vi "VersionDialog(CSM).vi"(7 "Name (\"\" to Use UUID)":string="Event CSM Tiny") -> ()   [LabVIEW 2020, in "CSMStand(Lite).lvlib"]
doc: "------------- lvcsm -------------\n[CSMStates]\nItem 0 = \"Event Structure\"\nItem 1 = \"Idle\"\nItem 2 = \"CSM Documentation\"\nItem 3 = \"VI Reference\"\nItem 4 = \"Error Handler\"\nItem 5 = \"Critical Error\"\nItem 6 = \"Target Error\"\nItem 7 = \"Target Timeout Error\"\nItem 8 = \"Async Response\"\nItem 9 = \"Response\"\nItem 10 = \"Async Message Posted\"\nItem 11 = \"Initialize Core Data\"\nItem 12 = \"Exit\"\nItem 13 = \"Data: Initialize\"\nItem 14 = \"Data: Cleanup\"\nItem 15 = \"Events: Register\"\nItem 16 = \"Events: Unregister\"\nItem 17 = \"UI: Initialize\"\nItem 18 = \"UI: Cursor Set\"\nItem 19 = \"UI: Front Panel State\"\nItem 20 = \"Macro: Initialize\"\nItem 21 = \"Macro: Exit\"\nItem 22 = \"API: API1\"\nItem 23 = \"API: API2\"\nItem 24 = \"Action: action1\"\nItem 25 = \"Action: action2\"\n\n[CSMStatus]\nItem 0 = \"Error Occurred@Error Handler\""
uses:
  CSMStand(Lite).lvlib
  <userlib>/_NEVSTOP/Communicable State Machine(CSM)/AdvanceAPI/CSM - Revert Arguments-Safe String.vi
  <userlib>/_NEVSTOP/Communicable State Machine(CSM)/AdvanceAPI/CSM - Make String Arguments Safe.vi
  <userlib>/_NEVSTOP/Communicable State Machine(CSM)/AdvanceAPI/CSM - Break Down Multiple States String.vi
  <userlib>/_NEVSTOP/Communicable State Machine(CSM)/AdvanceAPI/CSM - Compact Multiple States.vi
  <userlib>/_NEVSTOP/Communicable State Machine(CSM)/AdvanceAPI/CSM - Keywords.vi
  <userlib>/_NEVSTOP/Communicable State Machine(CSM)/_Shared/Trim Single-line Text.vi
  <userlib>/NEVSTOP-Programming-Palette/Dialog & Interface/Fit VI window to Visible Content_nevstop.vi
  <userlib>/_NEVSTOP/Communicable State Machine(CSM)/Communicable State Machine.lvlib
  <userlib>/_NEVSTOP/Communicable State Machine(CSM)/addons/API-String-Arugments-Support/API String Arguments Support.lvlib
panel:
  out "CSMVersion 2":string="Powered By CSM, Copyright ?2025 NEVSTOP-LAB"
  out "CSMStand(version) 2":string="CSMStand-Lite"
  out "CSMVersion":string
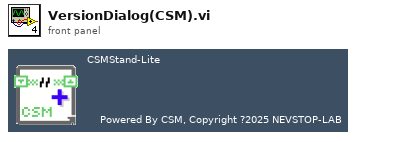
[diagram p1: front panel]
types:
  T1 = enum32{"Invalid", "Standard", "Closed", "Hidden", "Minimized", "Maximized"}
  T2 = enum32{"invalid app kind", "Development System", "Run Time System", "Student Edition", "Embedded LabVIEW", "Evaluation", "Custom"}
  T3 = typedef "Communicable State Machine.lvlib/_CSM_Response Source Message.ctl" = cluster{"‘State":string, "’Arguments":string, "’Error":errorcluster}
  T4 = cluster{"Current VI Reference":refnum<vi>, "Close Panel on Exit?":bool}
  T5 = cluster{"Core":cluster{"Current VI Reference":refnum<vi>, "Close Panel on Exit?":bool}, "Your Boolean data":bool, "Your string data":string}
  T6 = cluster{"Major":u16, "Minor":u16, "Fix":u16, "Build":u16}
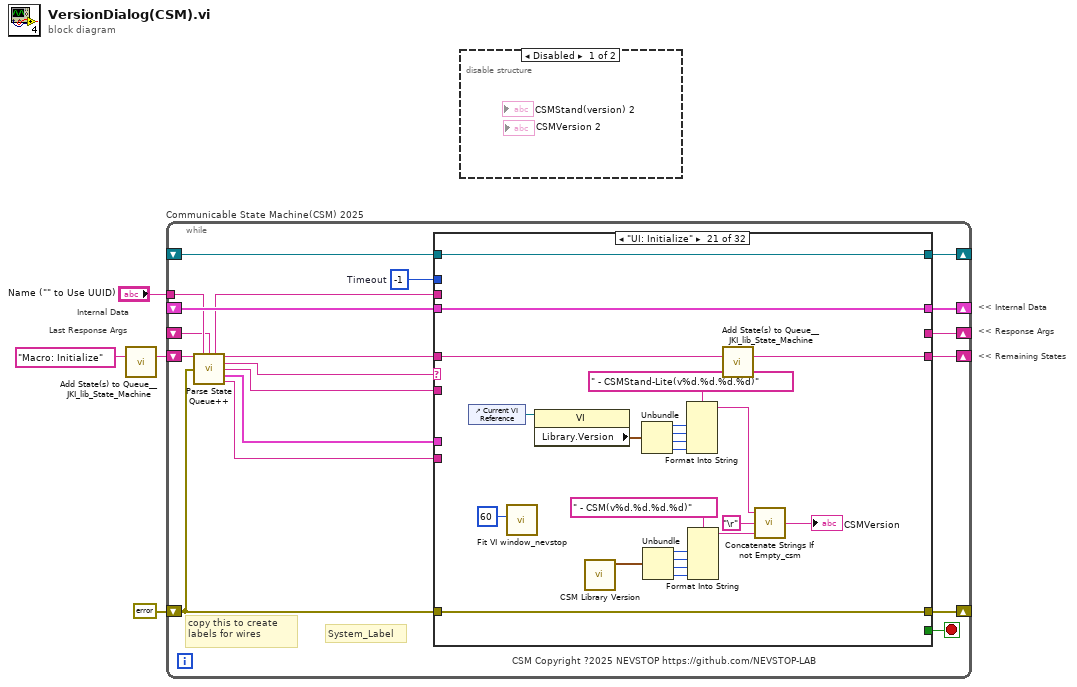
[diagram p0: block diagram]
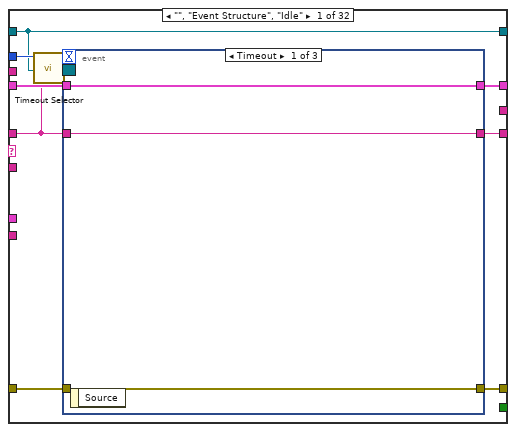
[diagram p3: hidden frame]
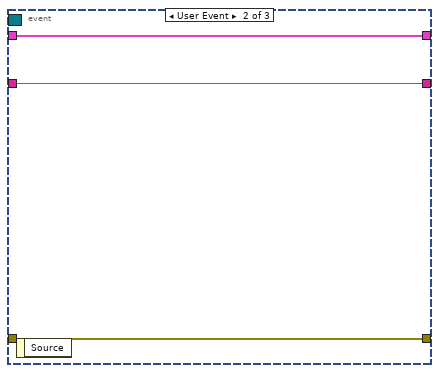
[diagram p4: hidden frame]
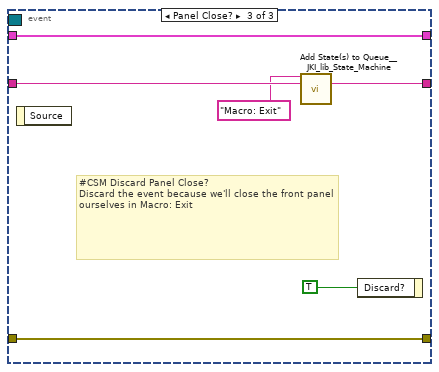
[diagram p5: hidden frame]
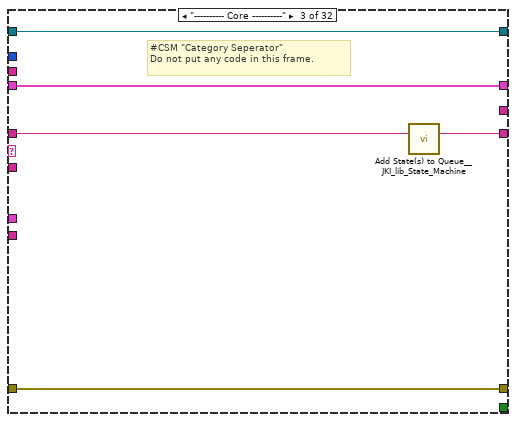
[diagram p7: hidden frame]
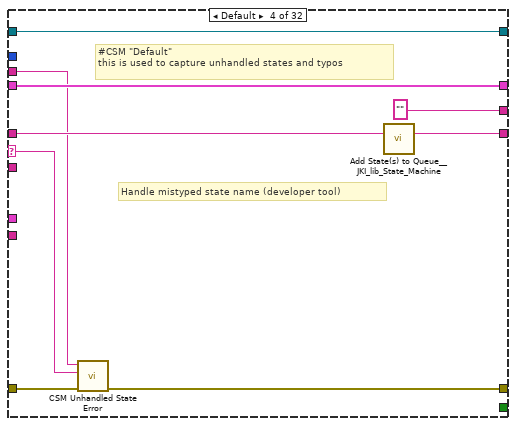
[diagram p8: hidden frame]
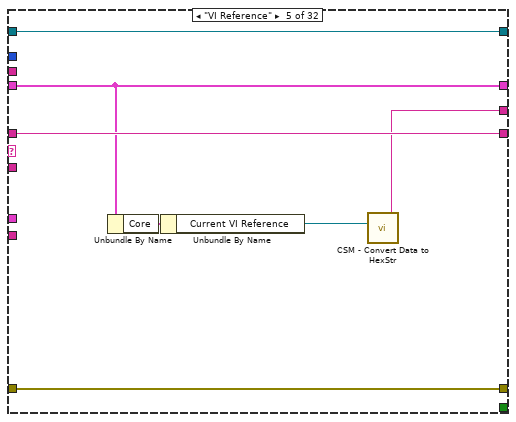
[diagram p9: hidden frame]
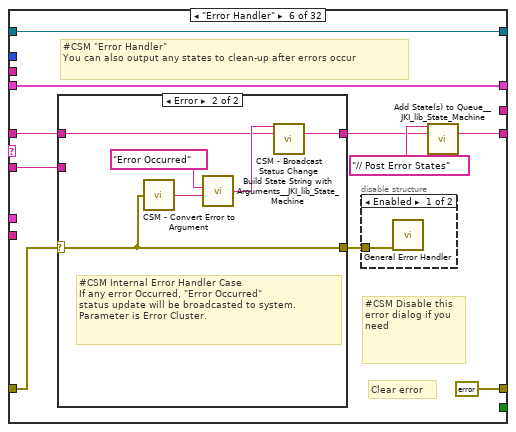
[diagram p10: hidden frame]
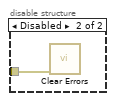
[diagram p11: hidden frame]
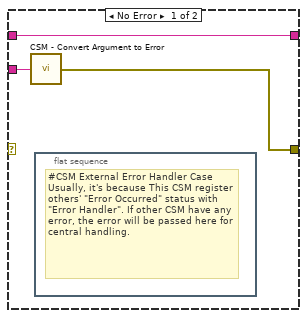
[diagram p12: hidden frame]
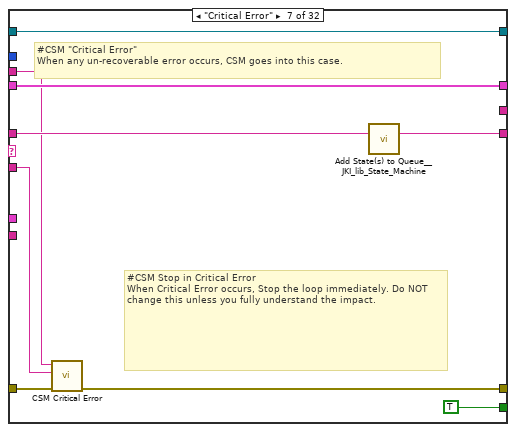
[diagram p13: hidden frame]
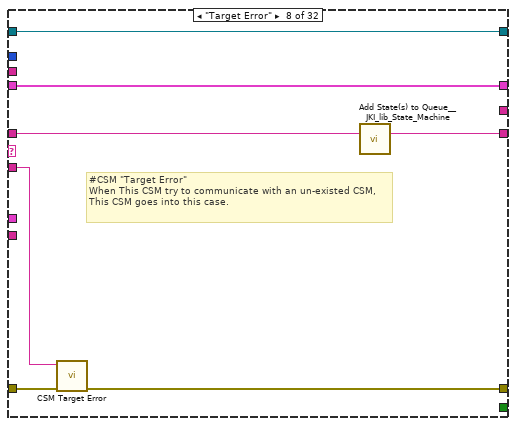
[diagram p14: hidden frame]
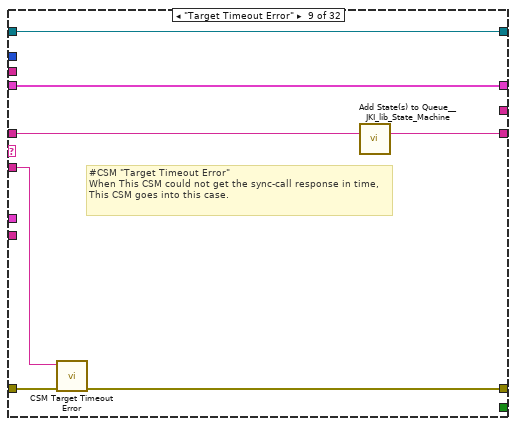
[diagram p15: hidden frame]
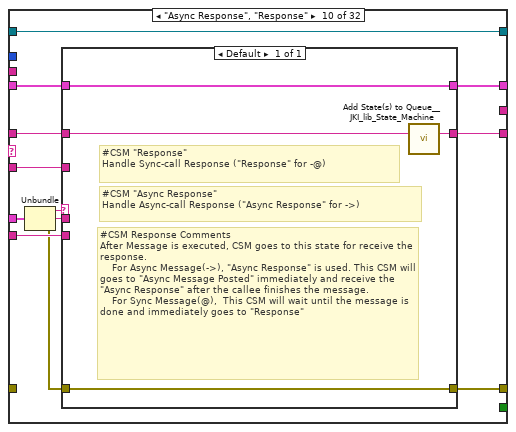
[diagram p16: hidden frame]
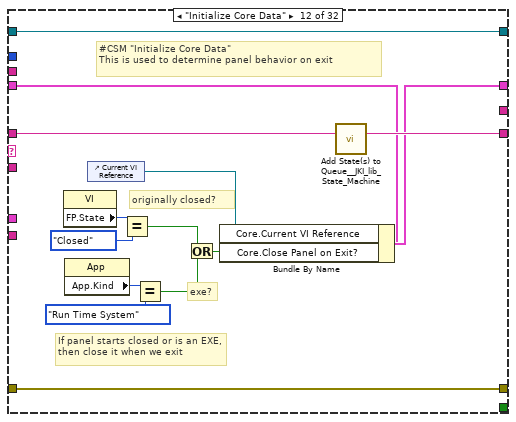
[diagram p18: hidden frame]
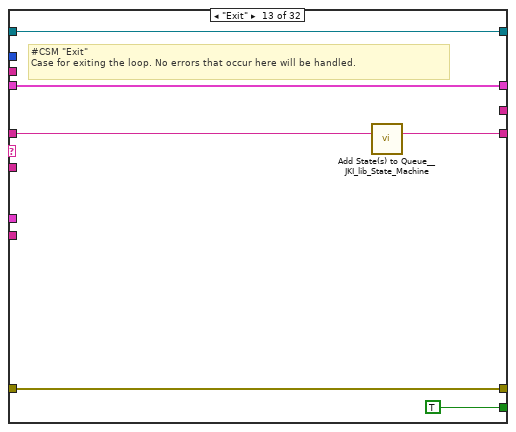
[diagram p19: hidden frame]
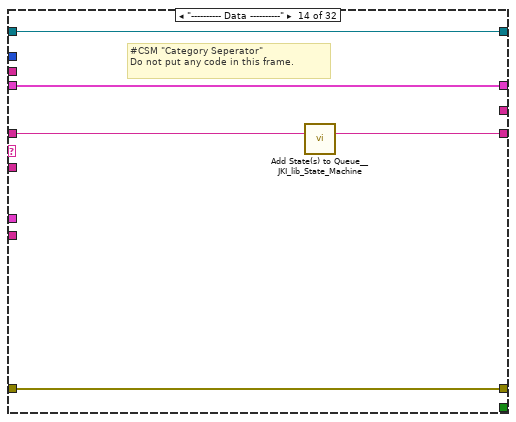
[diagram p20: hidden frame]
diagram:
  # "Last Response Args"
  # "Internal Data"
  # "<< Internal Data"
  # "<< Response Args"
  # "<< Remaining States"
  n1 = call <vilib>:"Add State(s) to Queue__JKI_lib_State_Machine.vi"("State(s) in (\"\")"="Macro: Initialize" ("Init State(\"Macro: Initialize\")")) -> ("States Out"=w1:string)  [unwired: 14 in]
  n2 = while "Communicable State Machine(CSM) 2025" {
    shift-right: [w18] -> _
    shift-left: _ -> [w17]
    shift-right: [w21] -> _
    shift-left: errorcluster {"status"=FALSE, "code"=0, "source"=""} ("error out") -> [w15]
    shift-right: [w20] -> _
    shift-left: w1 -> [w22]
    tunnel: "Name (\"\" to Use UUID)" -> [w11]
    shift-right: [w14] -> _
    shift-left: _ -> [w5]
    shift-right: [w13] -> _
    shift-left: _ -> [w12]
    stop <- w19 stop-if-true
    w16 = -1  # Timeout
    # "copy this to create labels for wires"
    # "System_Label"
    # "CSM Copyright ?2025 NEVSTOP https://github.com/NEVSTOP-LAB"
    n3 = call <userlib>:"Parse State Queue++.vi"("State Queue"=w22, "Name (\"\" to Use UUID)"=w11, "Response Arguments"=w5, "Previous Error"=w15) -> ("Name Used"=w6:string, "Remaining States"=w23:string, "Current State"=w10:string, "Arguments"=w9:string, "Additional Information"=w8:T3, "Source CSM"=w7:string)  [unwired: 6 in]
    n4 = case shown="\"UI: Initialize\"" w10 {
      selector: w10 -> [_ _ _ w56 _ _ _ _ _ _ _ _ _ _ _ _ _ _ _ _ _ _ _ _ _ _ _ _ _ _ _ _]
      tunnel: w23 -> [w24 w47 w53 w61 w68 w74 w97 w103 w110 w119 w132 w147 w153 w158 w166 w173 w178 w185 w189 w195 w218 w225 w241 w311 w317 w329 w332 w337 w343 w351 w356 w361]
      tunnel: w9 -> [_ _ _ _ _ w73 w92 w102 w109 w118 _ _ _ _ _ _ _ _ _ _ _ w220 w235 _ _ _ _ _ w340 _ _ _]
      tunnel: w17 -> [w31 w46 w50 w59 w67 w78 w98 w105 w112 w121 w131 w140 w151 w155 _ w168 w175 w184 w188 w192 w216 w223 w237 w308 w314 w326 w331 w336 w342 w348 w353 w358]
      tunnel: [w30 w48 w51 w54 w69 errorcluster {"status"=FALSE, "code"=0, "source"=""} ("error out") w93 w100 w107 w124 w133 w144 w150 w156 w163 w169 w176 w179 w187 w193 w215 w221 w238 w309 w315 w327 w333 w338 w344 w349 w354 w359] -> w21
      tunnel: w15 -> [w29 w48 w51 w62 w69 w75 w99 w101 w108 _ w133 w144 w150 w156 w163 w170 w176 _ w190 w193 w215 w222 w239 w309 w315 w327 w333 w338 w344 w349 w354 w359]
      tunnel: [w32 w47 w52 w60 w68 w70 w96 w106 w113 w120 w132 w146 w152 w157 w165 w172 w177 w185 w189 w194 w217 w224 w240 w310 w316 w328 w332 w337 w343 w350 w355 w360] -> w20
      tunnel: [_ _ _ _ _ _ TRUE _ _ _ _ _ TRUE _ _ _ _ _ _ _ _ _ _ _ _ _ _ _ _ _ _ _] -> w19
      tunnel: [w28 w46 w50 w59 w67 w78 w98 w105 w112 w122 w131 w145 w151 w155 w164 w168 w175 w184 w188 w192 w216 w223 w237 w308 w314 w326 w331 w336 w342 w348 w353 w358] -> w18
      tunnel: w16 -> [w27 _ _ _ _ _ _ _ _ _ _ _ _ _ _ _ _ _ _ _ _ _ _ _ _ _ _ _ _ _ _ _]
      tunnel: w7 -> [_ _ _ _ _ _ _ _ _ w116 _ _ _ _ _ _ _ _ _ _ _ _ _ _ _ _ _ _ _ _ _ _]
      tunnel: w8 -> [_ _ _ _ _ _ _ _ _ w123 _ _ _ _ _ _ _ _ _ _ _ _ _ _ _ _ _ _ _ _ _ _]
      tunnel: [_ _ _ "" w63 _ _ _ _ _ _ _ _ _ _ _ _ _ _ _ _ _ _ _ _ _ _ "API1 Response" w339 _ _ _] -> w14
      tunnel: [w26 w45 w49 w57 w66 w77 w94 w104 w111 w125 w130 w134 w148 w154 w159 w167 w174 w183 w186 w191 w214 w219 w234 w307 w312 w319 w330 w335 w341 w347 w352 w357] -> w13
      tunnel: w12 -> [w26 w45 w49 w57 w66 w77 w94 w104 w111 w125 w130 w134 w148 w154 w159 w167 w174 _ w186 w191 w214 w219 w234 w307 w312 w319 w330 w335 w341 w347 w352 w357]
      tunnel: w6 -> [_ _ _ w55 _ _ w91 _ _ _ _ _ _ _ _ _ _ w182 _ _ _ _ _ _ _ _ _ _ _ _ _ _]
      frame "", "Event Structure", "Idle" {
        n5 = call <userlib>:"Timeout Selector.vi"("Remaining States"=w24, "Timeout Expected"=w27) -> ("Timeout"=w25:i32)  [unwired: 5 in]
        n6 = event shown="[0] Timeout" {
          selector: w26 -> [_ _ _]
          dyn-events: _ -> [_ _ _]
          timeout: w25 -> [_ _ _]
          tunnel: w24 -> [w35 w37 w44]
          tunnel: [w35 w37 w43] -> w32
          tunnel: w31 -> [w33 w38 w41]
          tunnel: [w34 w36 w42] -> w30
          tunnel: w29 -> [w34 w36 w42]
          tunnel: [w33 w38 w41] -> w28
          event Timeout {
            n7 = event-data() -> ()  [unwired: 1 in, 1 out]
          }
          event User Event {
            n8 = event-data() -> ()  [unwired: 1 in, 1 out]
          }
          event Panel Close? {
            # "#CSM Discard Panel Close?\nDiscard the event because we'll close the front panel ourselves in Macro: Exit"
            n9 = event-data() -> ()  [unwired: 1 in, 1 out]
            n10 = call <vilib>:"Add State(s) to Queue__JKI_lib_State_Machine.vi"("State(s) in Front (\"\")"="Macro: Exit", "State(s) in (\"\")"=w44) -> ("States Out"=w43:string)  [unwired: 13 in]
            n11 = event-data("Discard?"=TRUE) -> ()  [unwired: 1 in, 1 out]
          }
        }
      }
      frame "CSM Documentation" {
      }
      frame "---------- Core ----------" {
        # "#CSM \"Category Seperator\"\nDo not put any code in this frame."
        n12 = call <vilib>:"Add State(s) to Queue__JKI_lib_State_Machine.vi"("State(s) in (\"\")"=w53) -> ("States Out"=w52:string)  [unwired: 14 in]
      }
      frame Default {
        # "#CSM \"Default\"\nthis is used to capture unhandled states and typos"
        # "Handle mistyped state name (developer tool)"
        n13 = call <userlib>:"CSM Unhandled State Error.vi"("error in (no error)"=w62, "Undefined State"=w56, "CSM Name"=w55) -> ("error out"=w54:errorcluster)  [unwired: 8 in]
        n14 = call <vilib>:"Add State(s) to Queue__JKI_lib_State_Machine.vi"("State(s) in (\"\")"=w61) -> ("States Out"=w60:string)  [unwired: 14 in]
      }
      frame "VI Reference" {
        n15 = Unbundle By Name(w67) -> ("Core"=w65:T4)
        n16 = Unbundle By Name(w65) -> ("Current VI Reference"=w64:refnum<vi>)
        n17 = call <userlib>:"CSM - Convert Data to HexStr.vi"("Variant"=w64) -> ("HEX String (0-9,A-F)"=w63:string)  [unwired: 8 in]
      }
      frame "Error Handler" {
        # "#CSM Disable this error dialog if you need"
        # "#CSM \"Error Handler\"\nYou can also output any states to clean-up after errors occur"
        # "Clear error"
        n18 = case shown="Error" w75 {
          selector: w75 -> [_ w85]
          tunnel: [w84 w87] -> w71
          tunnel: w74 -> [w84 w86]
          tunnel: w73 -> [w83 _]
          tunnel: [w82 w85] -> w76
          frame No Error {
            n19 = call <userlib>:"CSM - Convert Argument to Error.vi"("Argument"=w83) -> ("Error"=w82:errorcluster)  [unwired: 4 in]
            n20 = flat-sequence {
              frame #0 {
                # "#CSM External Error Handler Case\nUsually, it's because This CSM register others' \"Error Occurred\" status with \"Error Handler\". If other CSM have any error, the error will be passed here for central handling."
              }
            }
          }
          frame Error {
            # "#CSM Internal Error Handler Case \nIf any error Occurred, \"Error Occurred\" \nstatus update will be broadcasted to system.\nParameter is Error Cluster."
            n21 = call <userlib>:"CSM - Convert Error to Argument.vi"("Error"=w85) -> ("Argument"=w89:string)  [unwired: 4 in]
            n22 = call <vilib>:"Build State String with Arguments__JKI_lib_State_Machine.vi"("Arguments (\"\")"=w89, "State"="Error Occurred" ("Status with Arguments")) -> ("State with Arguments"=w88:string)  [unwired: 4 in]
            n23 = call <userlib>:"CSM - Broadcast Status Change.vi"("Status With Arguments"=w88, "State Queue"=w86) -> ("Remaining States"=w87:string)  [unwired: 13 in]
          }
        }
        n24 = disable-structure shown="Enabled" {
          disable-tunnel: w76 -> [w80 w81]
          frame Enabled {
            n25 = call <vilib>:"General Error Handler.vi"("error in (no error)"=w80) -> ()  [unwired: 10 in, 5 out]
          }
          frame Disabled {
            n26 = call <vilib>:"Clear Errors.vi"("error in (no error)"=w81) -> ()  [unwired: 5 in, 2 out]
          }
        }
        n27 = call <vilib>:"Add State(s) to Queue__JKI_lib_State_Machine.vi"("State(s) in Front (\"\")"="// Post Error States", "State(s) in (\"\")"=w71) -> ("States Out"=w70:string)  [unwired: 13 in]
      }
      frame "Critical Error" {
        # "#CSM Stop in Critical Error\nWhen Critical Error occurs, Stop the loop immediately. Do NOT change this unless you fully understand the impact."
        # "#CSM \"Critical Error\"\nWhen any un-recoverable error occurs, CSM goes into this case."
        n28 = call <userlib>:"CSM Critical Error.vi"("error in (no error)"=w99, "Arugments (As Reason)"=w92, "CSM Name"=w91) -> ("error out"=w93:errorcluster)  [unwired: 8 in]
        n29 = call <vilib>:"Add State(s) to Queue__JKI_lib_State_Machine.vi"("State(s) in (\"\")"=w97) -> ("States Out"=w96:string)  [unwired: 14 in]
      }
      frame "Target Error" {
        # "#CSM \"Target Error\"\nWhen This CSM try to communicate with an un-existed CSM, This CSM goes into this case."
        n30 = call <userlib>:"CSM Target Error.vi"("error in (no error)"=w101, "Arguments (As CSM Name)"=w102) -> ("error out"=w100:errorcluster)  [unwired: 9 in]
        n31 = call <vilib>:"Add State(s) to Queue__JKI_lib_State_Machine.vi"("State(s) in (\"\")"=w103) -> ("States Out"=w106:string)  [unwired: 14 in]
      }
      frame "Target Timeout Error" {
        # "#CSM \"Target Timeout Error\"\nWhen This CSM could not get the sync-call response in time, This CSM goes into this case."
        n32 = call <userlib>:"CSM Target Timeout Error.vi"("error in (no error)"=w108, "Arguments (As CSM Name)"=w109) -> ("error out"=w107:errorcluster)  [unwired: 9 in]
        n33 = call <vilib>:"Add State(s) to Queue__JKI_lib_State_Machine.vi"("State(s) in (\"\")"=w110) -> ("States Out"=w113:string)  [unwired: 14 in]
      }
      frame "Async Response", "Response" {
        n34 = Unbundle(w123) -> ("‘State"=w117:string, "’Arguments"=w115:string, "’Error"=w114:errorcluster)
        n35 = case shown="Default" w117 {
          tunnel: [w129] -> w124
          tunnel: w114 -> [w129]
          tunnel: [w128] -> w122
          tunnel: w121 -> [w128]
          tunnel: [w126] -> w120
          tunnel: w119 -> [w127]
          tunnel: w118 -> [_]
          tunnel: w116 -> [_]
          tunnel: w115 -> [_]
          frame Default {
            # "#CSM Response Comments\nAfter Message is executed, CSM goes to this state for receive the response.\n    For Async Message(->), \"Async Response\" is used. This CSM will goes to \"Async Message Posted\" immediately and receive the \"Async Response\" after the callee finishes the message.\n    For Sync Message(@),  This CSM will wait until the message is done and immediately goes to \"Response\""
            # "#CSM \"Async Response\"\nHandle Async-call Response (\"Async Response\" for ->)"
            # "#CSM \"Response\"\nHandle Sync-call Response (\"Response\" for -@)"
            n36 = call <vilib>:"Add State(s) to Queue__JKI_lib_State_Machine.vi"("State(s) in (\"\")"=w127) -> ("States Out"=w126:string)  [unwired: 14 in]
          }
        }
      }
      frame "Async Message Posted" {
        # "#CSM \"Async Message Posted\"\nAfter Async Message is posted (-> or ->| ), CSM goes to this state for post-action.\nYou can use Argument - State to tell which Async Message is called."
      }
      frame "Initialize Core Data" {
        # "#CSM \"Initialize Core Data\"\nThis is used to determine panel behavior on exit"
        # "originally closed?"
        # "exe?"
        # "If panel starts closed or is an EXE, then close it when we exit"
        n37 = property class="VI"() -> ("FP.State"=w137:T1)  [unwired: 2 in, 2 out]
        n38 = property class="App"() -> ("App.Kind"=w143:T2)  [unwired: 2 in, 2 out]
        n39 = control-ref of="Current VI Reference"() -> (w138:refnum<vi>)
        n40 = Equal?(x=w137, y=T1."Closed" ("Front Panel Window:State")) -> (x = y?=w135:bool)
        n41 = Equal?(x=w143, y=T2."Run Time System" ("Application:Kind")) -> (x = y?=w141:bool)
        n42 = Or(x=w135, y=w141) -> (x .or. y?=w139:bool)
        n43 = Bundle By Name(cluster=w140, "Core.Current VI Reference"=w138, "Core.Close Panel on Exit?"=w139) -> (w145:T5)
        n44 = call <vilib>:"Add State(s) to Queue__JKI_lib_State_Machine.vi"("State(s) in (\"\")"=w147) -> ("States Out"=w146:string)  [unwired: 14 in]
      }
      frame "Exit" {
        # "#CSM \"Exit\"\nCase for exiting the loop. No errors that occur here will be handled."
        n45 = call <vilib>:"Add State(s) to Queue__JKI_lib_State_Machine.vi"("State(s) in (\"\")"=w153) -> ("States Out"=w152:string)  [unwired: 14 in]
      }
      frame "---------- Data ----------" {
        # "#CSM \"Category Seperator\"\nDo not put any code in this frame."
        n46 = call <vilib>:"Add State(s) to Queue__JKI_lib_State_Machine.vi"("State(s) in (\"\")"=w158) -> ("States Out"=w157:string)  [unwired: 14 in]
      }
      frame "Data: Initialize" {
        w160 = T4 {"Current VI Reference"=refnum, "Close Panel on Exit?"=FALSE}  # Core
        w162 = TRUE  # Your Boolean data
        w161 = ""  # Your string data
        # "#CSM do not delete - used by framework"
        # "#CSM Expand Bundle to add new data elements to shift register data."
        # "#CSM Add new data here."
        # "Initialize the shift-register data, here.\n(data names are defined by what you wire into the bundle function)"
        n47 = Bundle("Core"=w160, "Your Boolean data"=w162, "Your string data"=w161) -> (w164:T5)  [unwired: 1 in]
        n48 = call <vilib>:"Add State(s) to Queue__JKI_lib_State_Machine.vi"("State(s) in (\"\")"=w166) -> ("States Out"=w165:string)  [unwired: 14 in]
      }
      frame "Data: Cleanup" {
        # "Cleanup any data and references, here.\n(this is called automatically, by the Macro: Exit)"
        n49 = Unbundle By Name(w168) -> ("Core.Current VI Reference"=w171:refnum<vi>)
        n50 = Close Reference(reference=w171, error in (no error)=w170) -> (error out=w169:errorcluster)
        n51 = call <vilib>:"Add State(s) to Queue__JKI_lib_State_Machine.vi"("State(s) in (\"\")"=w173) -> ("States Out"=w172:string)  [unwired: 14 in]
      }
      frame "---------- Events ----------" {
        # "#CSM \"Category Seperator\"\nDo not put any code in this frame."
        n52 = call <vilib>:"Add State(s) to Queue__JKI_lib_State_Machine.vi"("State(s) in (\"\")"=w178) -> ("States Out"=w177:string)  [unwired: 14 in]
      }
      frame "Events: Register" {
        # "#CSM \"Events: Register\"\nRegister user event. New Message Event is registered to break CSM waiting in event structure by default."
        # "#CSM Register New Message Event\nRegister message event to break Waiting in Event structure."
        n53 = call <userlib>:"CSM - Get New State Notifier Event.vi"("Name (\"\" to Use UUID)"=w182) -> ("error out"=w180:errorcluster, "New State Notifier Event"=w181:refnum<user-event>)  [unwired: 9 in]
        n54 = register-events(error in=w180, w181) -> (reference out=w183:refnum<event-registration>, error out=w179:errorcluster)  [unwired: 1 in]
      }
      frame "Events: Unregister" {
        # "#CSM \"Events: Unregister\"\nUnregister user event."
        n55 = Unregister For Events(event registration refnum=w186, error in=w190) -> (error out=w187:errorcluster)
      }
      frame "---------- UI ----------" {
        # "#CSM \"Category Seperator\"\nDo not put any code in this frame."
        n56 = call <vilib>:"Add State(s) to Queue__JKI_lib_State_Machine.vi"("State(s) in (\"\")"=w195) -> ("States Out"=w194:string)  [unwired: 14 in]
      }
      frame "UI: Initialize" {
        n57 = control-ref of="Current VI Reference"() -> (w213:refnum<vi>)
        n58 = call-poly <userlib>:"Fit VI window_nevstop.vi"("border spacing (2 px)"=60) -> ()  [unwired: 5 in, 2 out]
        n59 = property class="VI"(reference=w213) -> ("Library.Version"=w207:T6)  [unwired: 1 in, 2 out]
        n60 = call <userlib>:"CSM Library Version.vi"() -> ("Min-Compatible Version"=w201:T6)  [unwired: 10 in, 1 out]
        n61 = Unbundle(w207) -> ("Major"=w209:u16, "Minor"=w210:u16, "Fix"=w211:u16, "Build"=w212:u16)
        n62 = Unbundle(w201) -> ("Major"=w205:u16, "Minor"=w204:u16, "Fix"=w203:u16, "Build"=w202:u16)
        n63 = Format Into String(format string=" - CSMStand-Lite(v%d.%d.%d.%d)" ("String to Prepend to Source (\"\")"), w209, w210, w211, w212) -> (resulting string=w198:string)  [unwired: 2 in, 1 out]
        n64 = Format Into String(format string=" - CSM(v%d.%d.%d.%d)" ("String to Prepend to Source (\"\")"), w205, w204, w203, w202) -> (resulting string=w197:string)  [unwired: 2 in, 1 out]
        n65 = call <vilib>:"Add State(s) to Queue__JKI_lib_State_Machine.vi"("State(s) in (\"\")"=w218) -> ("States Out"=w217:string)  [unwired: 14 in]
        n66 = call <userlib>:"Concatenate Strings If not Empty_csm.vi"("String"=w197, "seperator(:)"="\r", "prefix"=w198) -> ("result"=→"CSMVersion":string)  [unwired: 2 in]
      }
      frame "UI: Cursor Set" {
        # "#CSM \"UI: Cursor Set\"\nSet and Unset Cursor Busy.\n(Usage: \"UI: Cursor Set >> Busy|Idle\")"
        # "Argument"
        n67 = disable-structure shown="Default" {
          disable-tunnel: w222 -> [w228 w233]
          disable-tunnel: [w227 w233] -> w221
          disable-tunnel: w220 -> [w226 _]
          frame condition #0 (active) {
            n68 = case shown="\"Idle\", Default" w226 {
              tunnel: w228 -> [w230 w232]
              tunnel: [w229 w231] -> w227
              frame "Idle", Default {
                n69 = call <vilib>:"Unset Busy.vi"("error in (no error)"=w230) -> ("error out"=w229:errorcluster)  [unwired: 10 in]
              }
              frame "Busy" {
                n70 = call <vilib>:"Set Busy.vi"("error in (no error)"=w232) -> ("error out"=w231:errorcluster)  [unwired: 9 in, 1 out]
              }
            }
          }
          frame condition #1 {
          }
        }
        n71 = call <vilib>:"Add State(s) to Queue__JKI_lib_State_Machine.vi"("State(s) in (\"\")"=w225) -> ("States Out"=w224:string)  [unwired: 14 in]
      }
      frame "UI: Front Panel State" {
        # "#CSM \"UI: Front Panel State\"\nSet Front Panel Open or Closed\n(Usage: \"UI: Front Panel State >> Open|Close\")"
        # "Argument"
        n72 = Unbundle By Name(w237) -> ("Core.Current VI Reference"=w236:refnum<vi>)
        n73 = call <vilib>:"Add State(s) to Queue__JKI_lib_State_Machine.vi"("State(s) in (\"\")"=w241) -> ("States Out"=w240:string)  [unwired: 14 in]
        n74 = case shown="\"Close\", \"Closed\"" w235 {
          tunnel: w239 -> [w247 w262 w273 w286 w299]
          tunnel: [w249 w263 w275 w288 w301] -> w238
          tunnel: w236 -> [w248 w260 w274 w287 w300]
          frame "Open", "Standard", Default {
            w242 = T1."Standard" ("State")
            n75 = property class="VI"(reference=w248, error in=w247) -> (reference out=w245:refnum<vi>, error out=w246:errorcluster, "FP.State"=w244:T1)
            n76 = Not Equal?(x=w244, y=w242) -> (x != y?=w243:bool)
            n77 = case shown="True" w243 {
              tunnel: [w253 w255] -> w249
              tunnel: w246 -> [w252 w255]
              tunnel: w245 -> [w251 _]
              tunnel: w242 -> [w250 _]
              frame True {
                n78 = invoke class="VI" method="FP.Open"(reference=w251, error in=w252, "Activate"=TRUE, "State"=w250) -> (error out=w253:errorcluster)  [unwired: 1 in, 4 out]
              }
              frame False {
              }
            }
          }
          frame "Close", "Closed" {
            n79 = property class="VI"(reference=w260, error in=w262) -> (reference out=w259:refnum<vi>, error out=w261:errorcluster, "FP.State"=w257:T1)
            n80 = Not Equal?(x=w257, y=T1."Closed" ("Front Panel Window:State")) -> (x != y?=w256:bool)
            n81 = case shown="False" w256 {
              tunnel: [w264 w267] -> w263
              tunnel: w261 -> [w264 w266]
              tunnel: w259 -> [_ w265]
              frame False {
              }
              frame True {
                n82 = invoke class="VI" method="FP.Close"(reference=w265, error in=w266) -> (error out=w267:errorcluster)  [unwired: 1 in, 2 out]
              }
            }
          }
          frame "Hidden", "Hide" {
            w268 = T1."Hidden" ("State")
            n83 = property class="VI"(reference=w274, error in=w273) -> (reference out=w271:refnum<vi>, error out=w272:errorcluster, "FP.State"=w270:T1)
            n84 = Not Equal?(x=w270, y=w268) -> (x != y?=w269:bool)
            n85 = case shown="True" w269 {
              tunnel: [w279 w280] -> w275
              tunnel: w272 -> [w278 w280]
              tunnel: w271 -> [w277 _]
              tunnel: w268 -> [w276 _]
              frame True {
                n86 = invoke class="VI" method="FP.Open"(reference=w277, error in=w278, "State"=w276) -> (error out=w279:errorcluster)  [unwired: 2 in, 4 out]
              }
              frame False {
              }
            }
          }
          frame "Minimize", "Minimized" {
            w281 = T1."Minimized" ("State")
            n87 = property class="VI"(reference=w287, error in=w286) -> (reference out=w284:refnum<vi>, error out=w285:errorcluster, "FP.State"=w283:T1)
            n88 = Not Equal?(x=w283, y=w281) -> (x != y?=w282:bool)
            n89 = case shown="True" w282 {
              tunnel: [w292 w293] -> w288
              tunnel: w285 -> [w291 w293]
              tunnel: w284 -> [w290 _]
              tunnel: w281 -> [w289 _]
              frame True {
                n90 = invoke class="VI" method="FP.Open"(reference=w290, error in=w291, "State"=w289) -> (error out=w292:errorcluster)  [unwired: 2 in, 4 out]
              }
              frame False {
              }
            }
          }
          frame "Maximize", "Maximized" {
            w294 = T1."Maximized" ("State")
            n91 = property class="VI"(reference=w300, error in=w299) -> (reference out=w297:refnum<vi>, error out=w298:errorcluster, "FP.State"=w296:T1)
            n92 = Not Equal?(x=w296, y=w294) -> (x != y?=w295:bool)
            n93 = case shown="True" w295 {
              tunnel: [w305 w306] -> w301
              tunnel: w298 -> [w304 w306]
              tunnel: w297 -> [w303 _]
              tunnel: w294 -> [w302 _]
              frame True {
                n94 = invoke class="VI" method="FP.Open"(reference=w303, error in=w304, "State"=w302) -> (error out=w305:errorcluster)  [unwired: 2 in, 4 out]
              }
              frame False {
              }
            }
          }
        }
      }
      frame "---------- Macro ----------" {
        # "#CSM \"Category Seperator\"\nDo not put any code in this frame."
        n95 = call <vilib>:"Add State(s) to Queue__JKI_lib_State_Machine.vi"("State(s) in (\"\")"=w311) -> ("States Out"=w310:string)  [unwired: 14 in]
      }
      frame "Macro: Initialize" {
        w313 = "Data: Initialize\nInitialize Core Data\nEvents: Register\nUI: Initialize\n//UI: Front Panel State >> Open"  # Data: Initialize Initialize Core Data Events: Register UI: Initialize //UI: Front Panel State >> Open
        # "#CSM \"Macro: Initialize\"\nInitialization Macro (This is called once, when the VI starts)"
        n96 = call <vilib>:"Add State(s) to Queue__JKI_lib_State_Machine.vi"("State(s) in Front (\"\")"=w313, "State(s) in (\"\")"=w317) -> ("States Out"=w316:string)  [unwired: 13 in]
      }
      frame "Macro: Exit" {
        # "#CSM \"Macro: Exit\"\nExit Macro (This is called once, when the VI exits)"
        n97 = Unbundle By Name(w326) -> ("Core.Close Panel on Exit?"=w325:bool)
        n98 = Select(t="UI: Front Panel State >> Close", s=w325, f="") -> (s? t:f=w322:string)
        n99 = call <vilib>:"Add State(s) to Queue__JKI_lib_State_Machine.vi"("State(s) in Front (\"\")"="//Exit Sub-Modules ", "State(s) in (\"\")"=w322, "State(s) at Back (\"\")"="Data: Cleanup\nEvents: Unregister\nExit") -> ("States Out"=w320:string)  [unwired: 12 in]
        n100 = call <vilib>:"Add State(s) to Queue__JKI_lib_State_Machine.vi"("State(s) in Front (\"\")"=w320, "State(s) in (\"\")"=w329) -> ("States Out"=w328:string)  [unwired: 13 in]
      }
      frame "---------- API ----------" {
        # "#CSM \"Category Seperator\"\nDo not put any code in this frame."
      }
      frame "API: API1" {
        # "#CSM API Example\nCopy/Rename this case for your own API"
        # "#CSM Response\nConnect this to return the response of your API"
        # "#CSM >> Source CSM >>\nIf you need to tell who triggered this state , use this string. If it's this case itself, this string is \"\"."
        # "#CSM >> Arguments >>\nDeal with the parameter if any"
      }
      frame "API: API2" {
        # "#CSM API Example\nCopy/Rename this case for your own API"
        # "unpack Hex String  to Variant\nif complex parameter is needed."
        n101 = call <userlib>:"CSM - Convert HexStr to Data.vi"("HEX String"=w340) -> ()  [unwired: 7 in, 2 out]
        n102 = disable-structure shown="Disabled" {
          disable-tunnel: [w345 "API2 Response"] -> w339
          frame Disabled {
            # "pack variant to hexstr \nif complex response is needed."
            # "complex Response"
            n103 = call <userlib>:"CSM - Convert Data to HexStr.vi"() -> ("HEX String (0-9,A-F)"=w345:string)  [unwired: 9 in]
          }
          frame Enabled {
          }
        }
      }
      frame "---------- Action ----------" {
        # "#CSM \"Category Seperator\"\nDo not put any code in this frame."
        n104 = call <vilib>:"Add State(s) to Queue__JKI_lib_State_Machine.vi"("State(s) in (\"\")"=w351) -> ("States Out"=w350:string)  [unwired: 14 in]
      }
      frame "Action: action1" {
        # "#CSM \"Internal State\"\nThis category is used for holding internal states"
        n105 = call <vilib>:"Add State(s) to Queue__JKI_lib_State_Machine.vi"("State(s) in (\"\")"=w356) -> ("States Out"=w355:string)  [unwired: 14 in]
      }
      frame "Action: action2" {
        # "#CSM \"Internal State\"\nThis category is used for holding internal states"
        n106 = call <vilib>:"Add State(s) to Queue__JKI_lib_State_Machine.vi"("State(s) in (\"\")"=w361) -> ("States Out"=w360:string)  [unwired: 14 in]
      }
    }
  }
  n107 = disable-structure shown="Disabled" {
    frame Disabled {
    }
    frame Enabled {
    }
  }
